vi "find team's alliance scores.vi"(0 "Data sources":path[](array[path]), 3 "seeding data":T1={"read seed value from file"=FALSE, "seed source file path"=path "", "indexes"={"index"=2, "index 2"=3}, "subtract from"=0.0}) -> (1 "team/match locator":i16[][](array[numeric]), 2 "Array":T2(array[cluster]), 4 "alliance info":i16[][](array[numeric]), 5 "team scoring OK?":bool)   [LabVIEW 2009]
uses:
  <vilib>/Utility/file.llb/Read From Spreadsheet File (I64).vi
  <vilib>/Utility/file.llb/Read From Spreadsheet File (DBL).vi
  <vilib>/Analysis/NI_AALBase.lvlib
panel:
  in  "data soure file path":path
  out "x = y?":bool
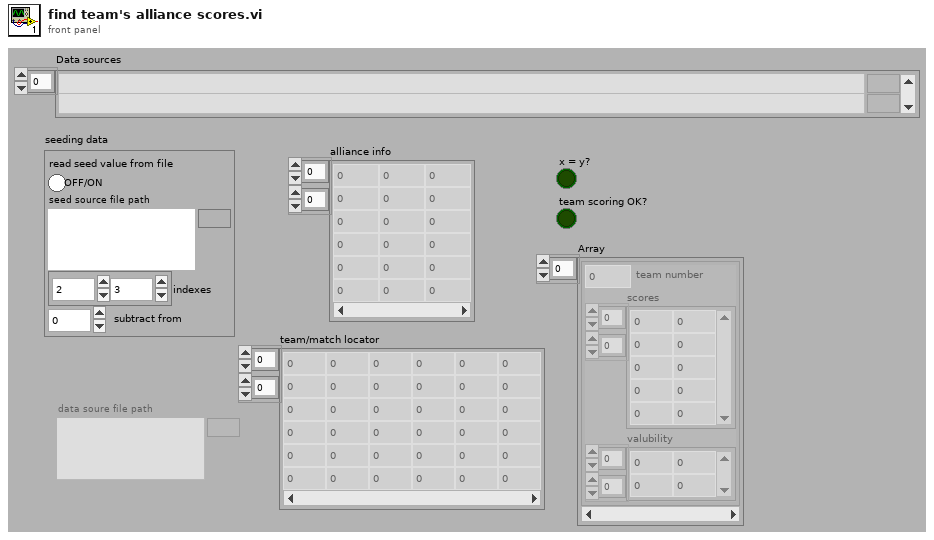
[diagram p1: front panel]
types:
  T1 = cluster{"read seed value from file":bool, "seed source file path":path, "indexes":cluster{"index":i32, "index 2":i32}, "subtract from":dbl}
  T2 = cluster{i16, "scores":i16[][], "valubility":dbl[][]}[]
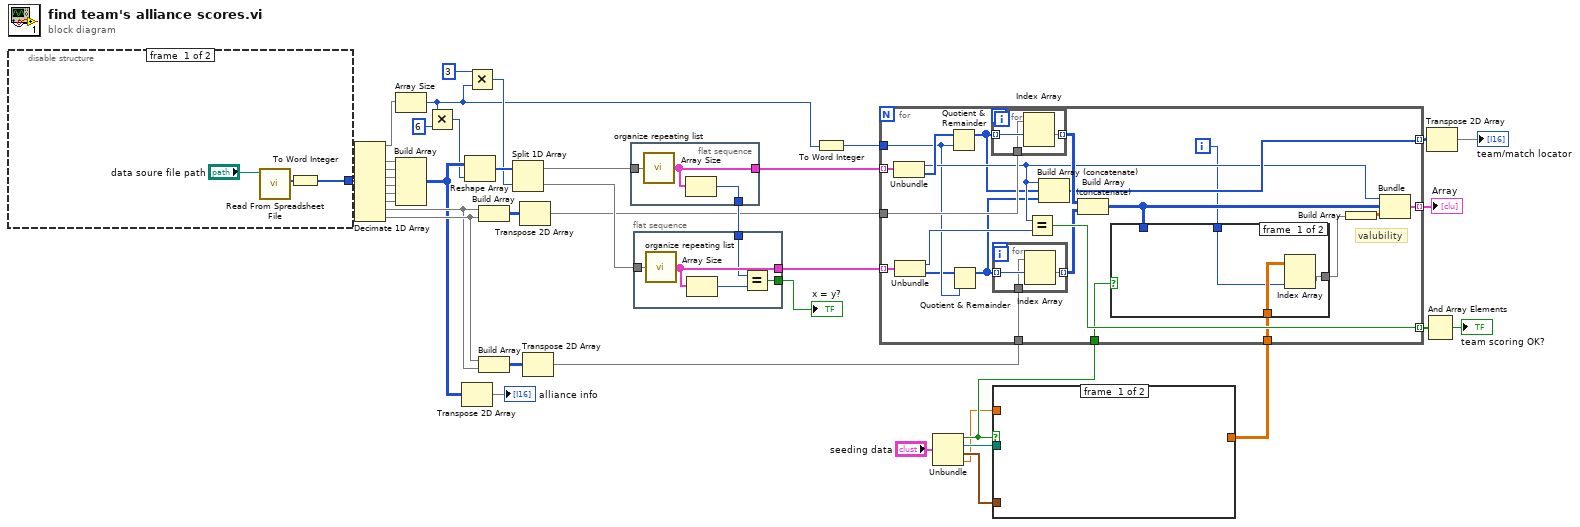
[diagram p0: block diagram]
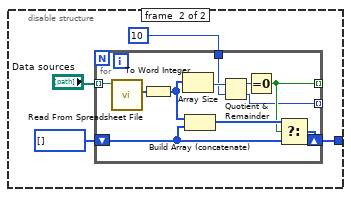
[diagram p2: hidden frame]
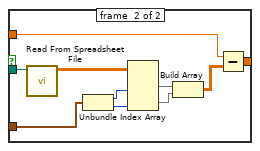
[diagram p3: hidden frame]
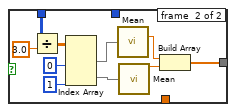
[diagram p4: hidden frame]
diagram:
  n1 = disable-structure shown="Enabled" {
    disable-tunnel: [w41 w44] -> w31
    frame #0 {
      n2 = call-poly <vilib>:"Read From Spreadsheet File.vi"("file path (dialog if empty)"="data soure file path") -> ("first row"=w43:i64[])  [unwired: 6 in, 4 out]
      n3 = To Word Integer(number=w43) -> (16bit integer=w41:i16[])
    }
    frame #1 {
      n4 = for {
        tunnel: "Data sources" -> [w58] mode=indexing
        shift-right: [w51] -> w44
        shift-left: i16[] [] -> [w50]
        tunnel: 10 -> [w54]
        tunnel: [w49] -> _ mode=indexing
        tunnel: [w48] -> _ mode=indexing
        n5 = call-poly <vilib>:"Read From Spreadsheet File.vi"("file path (dialog if empty)"=w58) -> ("first row"=w57:i64[])  [unwired: 6 in, 4 out]
        n6 = To Word Integer(number=w57) -> (16bit integer=w56:i16[])
        n7 = Array Size(array=w56) -> (size(s)=w55:i32)
        n8 = Build Array (concatenate)(w56, w50) -> (w52:i16[])
        n9 = Quotient & Remainder(x=w55, y=w54) -> (x-y*floor(x/y)=w53:i32, floor(x/y)=w48:i32)
        n10 = Equal To 0?(x=w53) -> (x = 0?=w49:bool)
        n11 = Select(t=w52, s=w49, f=w50) -> (s? t:f=w51:i16[])
      }
    }
  }
  n12 = Decimate 1D Array(w31) -> (w15:i16[], w25:i16[], w26:i16[], w27:i16[], w28:i16[], w29:i16[], w30:i16[], w39:i16[], w40:i16[])  [unwired: 1 out]
  n13 = Array Size(array=w15) -> (size(s)=w8:i32)
  n14 = Build Array(w25, w26, w27, w28, w29, w30) -> (w24:i16[][])
  n15 = Multiply(x=w8, y=6) -> (x*y=w19:i32)
  n16 = Transpose 2D Array(2D array=w24) -> (transposed array=→"alliance info":i16[][])
  n17 = Reshape Array(w24, w19) -> (w23:i16[])
  n18 = Multiply(x=3 ("y"), y=w8) -> (x*y=w17:i32)
  n19 = Build Array(w39, w40) -> (w38:i16[][])
  n20 = Build Array(w40, w39) -> (w14:i16[][])
  n21 = Split 1D Array(array=w23, index=w17) -> (first subarray=w22:i16[], second subarray=w21:i16[])
  n22 = Transpose 2D Array(2D array=w38) -> (transposed array=w16:i16[][])
  n23 = Transpose 2D Array(2D array=w14) -> (transposed array=w13:i16[][])
  n24 = flat-sequence {
    tunnel: w22 -> [w61]
    tunnel: [w60] -> w37
    tunnel: [w59] -> w35
    frame #0 {
      n25 = call "organize repeating list.vi"("Array in"=w61) -> ("Array out"=w60:cluster{i16, i32[]}[])
      n26 = Array Size(array=w60) -> (size(s)=w59:i32)
    }
  }
  n27 = flat-sequence {
    tunnel: w21 -> [w66]
    tunnel: [w65] -> w36
    tunnel: w35 -> [w64]
    tunnel: [w62] -> w32
    frame #0 {
      n28 = call "organize repeating list.vi"("Array in"=w66) -> ("Array out"=w65:cluster{i16, i32[]}[])
      n29 = Array Size(array=w65) -> (size(s)=w63:i32)
      n30 = Equal?(x=w64, y=w63) -> (x = y?=w62:bool)
    }
  }
  n31 = To Word Integer(number=w8) -> (16bit integer=w7:i16)
  n32 = Unbundle("seeding data") -> ("read seed value from file"=w4:bool, "seed source file path"=w3:path, "indexes"=w2:cluster{"index":i32, "index 2":i32}, "subtract from"=w1:dbl)
  n33 = case shown="True" w4 {
    tunnel: w3 -> [_ w76]
    tunnel: [_ w68] -> w6
    tunnel: w2 -> [_ w70]
    tunnel: w1 -> [_ w69]
    frame #0 {
    }
    frame #1 {
      n34 = call-poly <vilib>:"Read From Spreadsheet File.vi"("file path (dialog if empty)"=w76) -> ("all rows"=w75:dbl[][])  [unwired: 6 in, 4 out]
      n35 = Unbundle(w70) -> ("index"=w73:i32, "index 2"=w74:i32)
      n36 = Index Array(array=w75, index (col) #1=w73, index (col) #2=w74) -> (element #1=w72:dbl[], element #2=w71:dbl[])  [unwired: 2 in]
      n37 = Build Array(w72, w71) -> (w67:dbl[][])
      n38 = Subtract(x=w69, y=w67) -> (x-y=w68:dbl[][])
    }
  }
  n39 = for {
    tunnel: w37 -> [w98] mode=indexing
    tunnel: w7 -> [w84]
    tunnel: w16 -> [w97]
    tunnel: w36 -> [w96] mode=indexing
    tunnel: w13 -> [w95]
    tunnel: [w93] -> w12 mode=indexing
    tunnel: [w86] -> w34 mode=indexing
    tunnel: [w91] -> w11 mode=indexing
    tunnel: w4 -> [w80]
    tunnel: w6 -> [w79]
    i -> [w77]
    # "valubility"
    n40 = Unbundle(w98) -> (w85:i16, w87:i32[])
    n41 = Unbundle(w96) -> (w92:i16, w81:i32[])
    n42 = Quotient & Remainder(x=w87, y=w84) -> (x-y*floor(x/y)=w83:i32[])  [unwired: 1 out]
    n43 = Quotient & Remainder(x=w81, y=w84) -> (x-y*floor(x/y)=w82:i32[])  [unwired: 1 out]
    n44 = for {
      tunnel: w83 -> [w117] mode=indexing
      tunnel: w97 -> [w116]
      tunnel: [w115] -> w94 mode=indexing
      n45 = Index Array(array=w116, index (row)=w117) -> (element=w115:i16[])  [unwired: 1 in]
    }
    n46 = for {
      tunnel: w82 -> [w114] mode=indexing
      tunnel: [w113] -> w78 mode=indexing
      tunnel: w95 -> [w112]
      n47 = Index Array(array=w112, index (row)=w114) -> (element=w113:i16[])  [unwired: 1 in]
    }
    n48 = Equal?(x=w85, y=w92) -> (x = y?=w86:bool)
    n49 = Build Array (concatenate)(w85, w83, w82) -> (w91:i32[])
    n50 = Build Array (concatenate)(w94, w78) -> (w90:i16[][])
    n51 = case shown="False" w80 {
      tunnel: w90 -> [_ w109]
      tunnel: [w101 w102] -> w89
      tunnel: w79 -> [w100 _]
      tunnel: w77 -> [w99 _]
      frame #0 {
        n52 = Index Array(array=w100, index (col)=w99) -> (element=w101:dbl[])  [unwired: 1 in]
      }
      frame #1 {
        n53 = Divide(x=w109, y=3.0) -> (x/y=w110:dbl[][])
        n54 = Index Array(array=w110, index (col) #1=0 ("disabled index (col)"), index (col) #2=1 ("index (col)")) -> (element #1=w106:dbl[], element #2=w105:dbl[])  [unwired: 2 in]
        n55 = call <vilib>:"Mean.vi"("X"=w106) -> ("mean"=w103:dbl)  [unwired: 1 out]
        n56 = call <vilib>:"Mean.vi"("X"=w105) -> ("mean"=w104:dbl)  [unwired: 1 out]
        n57 = Build Array(w103, w104) -> (w102:dbl[])
      }
    }
    n58 = Build Array(w89) -> (w88:dbl[][])
    n59 = Bundle(w85, w90, w88) -> (w93:cluster{i16, i16[][], dbl[][]})  [unwired: 1 in]
  }
  "Array" <- w12
  n60 = And Array Elements(Boolean array=w34) -> (logical AND=→"team scoring OK?":bool)
  n61 = Transpose 2D Array(2D array=w11) -> (transposed array=→"team/match locator":i32[][])
  "x = y?" <- w32
